vi "Get Access Token.vi"(8 "Error In (No Error)":errorcluster) -> (1 "token response (JSON)":string, 2 "access token":string caption="<JSON>Item")   [LabVIEW 2019, in "Useful OAuth VIs.lvlib"]
uses:
  Useful OAuth VIs.lvlib
  e7adaa82-728e-4af2-911a-35986e5cd437.vi
  2f0a06cf-a99b-4825-b433-179a9c98a469.vi
  <vilib>/JDP Science/JSONtext/Find Item.vi
  <vilib>/JDP Science/JSONtext/String Subset.vi
  globals.vi
  <vilib>/httpClient/POSTBuffer.vi
  <vilib>/JDP Science/JSONtext/Parsing/Parse Full Path or Item Name.vi
  <vilib>/JDP Science/JSONtext/Next JSON Value.vi
  <vilib>/JDP Science/JSONtext/support/Error Cluster From Code.vi
  <vilib>/JDP Science/JSONtext/Offset/Find Item Locations by Path.vi
  <vilib>/JDP Science/JSONtext/JSON text to Variant.vi
  <vilib>/JDP Science/JSONtext/LVClass Serializer/JSONtext LVClass Serializer.lvclass
  <vilib>/httpClient/LabVIEWHTTPClient.lvlib
  <vilib>/wsapi/NI_WebServices.lvlib
panel:
  out "error out":errorcluster
  in  "Redirect URI":string="http://localhost:8001/OAuth/Redirect"
  in  "Client Secret":string="Tx~D4BO32ip_x~_salD8.nHFyC7XIXCKuI"
  in  "Scopes (separated by single space)":string="offline_access Notes.ReadWrite"
  in  "Client ID":string="6224e1bc-8db0-4ef6-9504-7e49f93fdd78"
  in  "Tenant Type":string="organizations"
  out "Request body":string
  out "Request URI":string
  out "headers":string
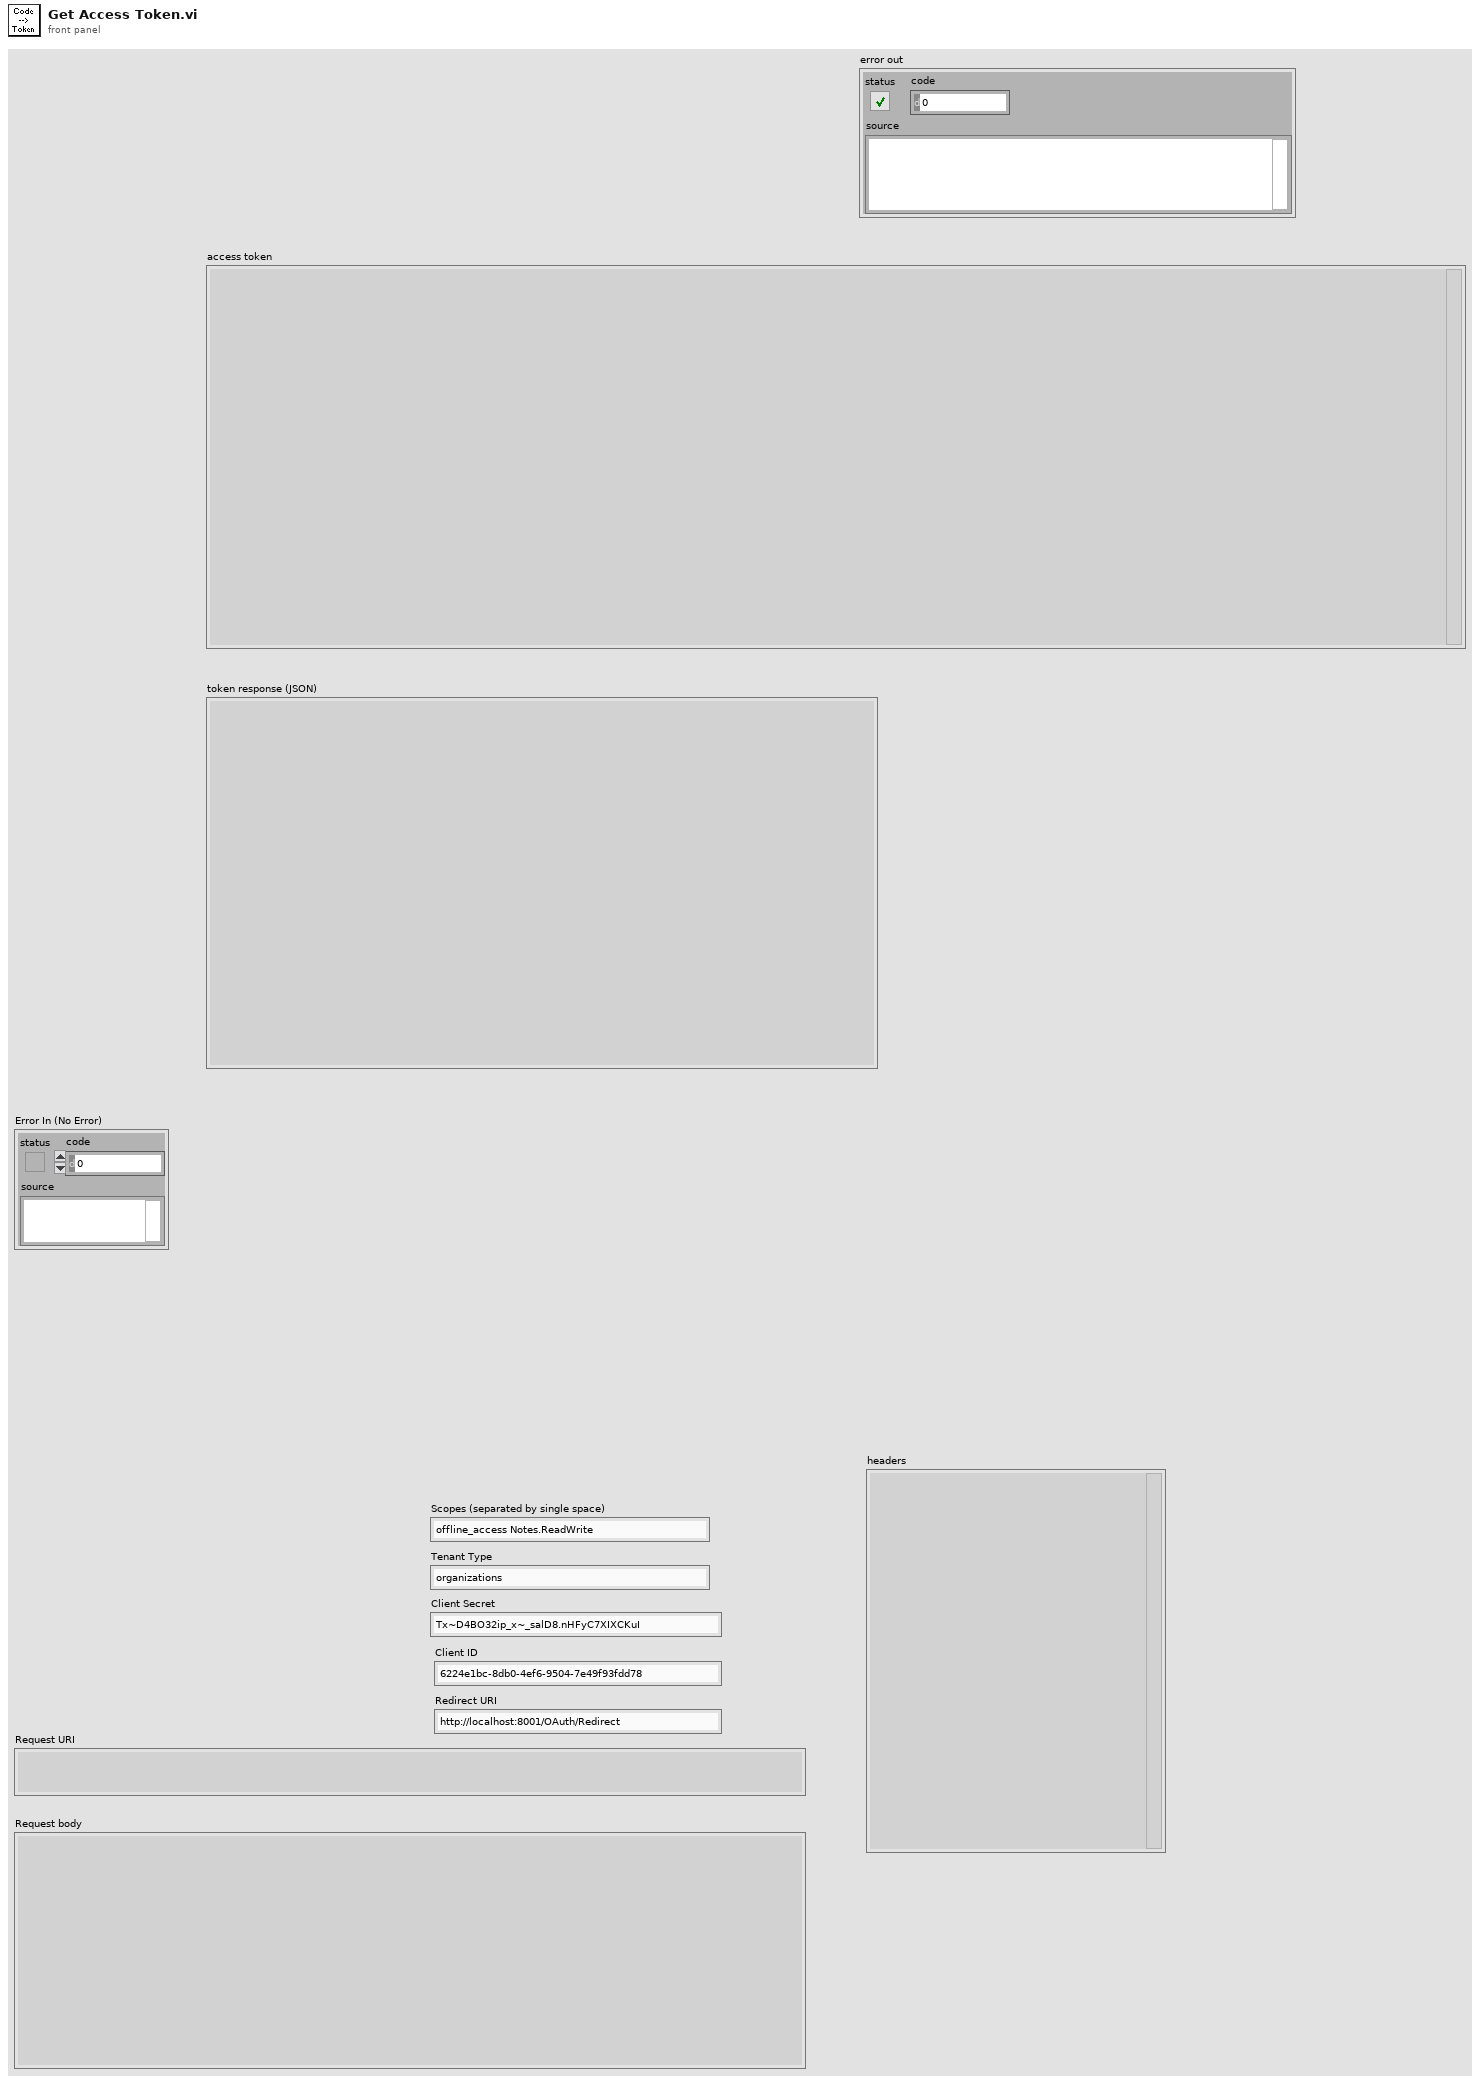
[diagram p1: front panel]
types:
  T1 = typedef "LabVIEWHTTPClient.lvlib/ClientHandle.ctl" = refnum<k1>
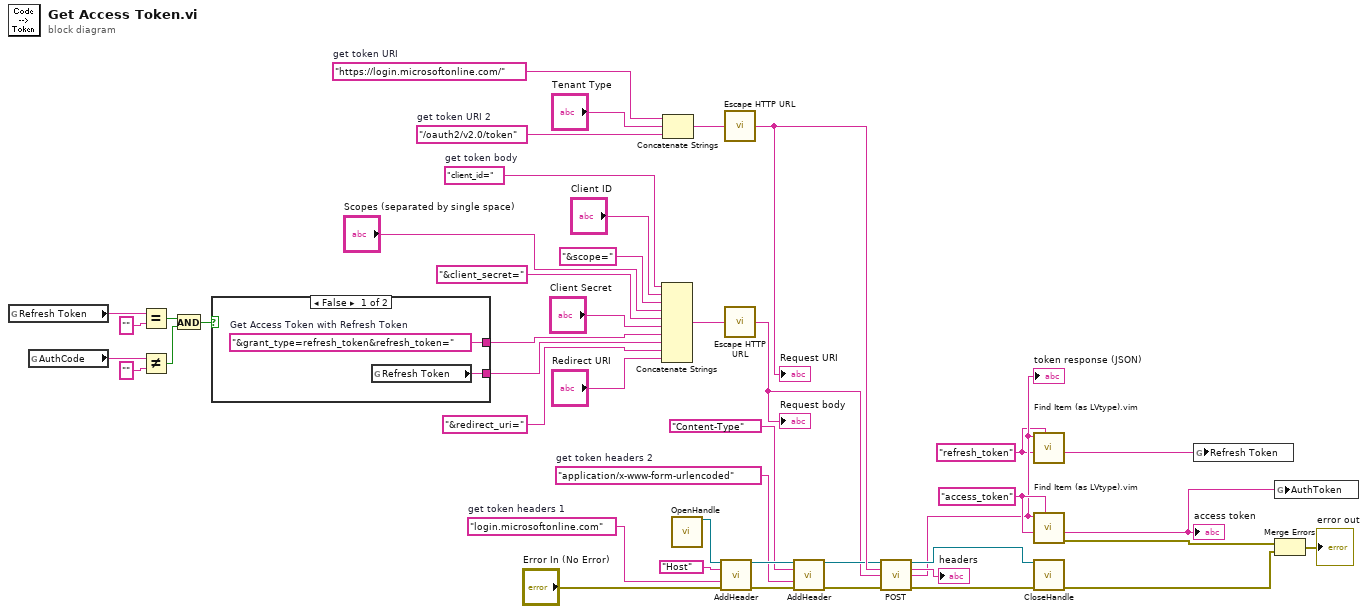
[diagram p0: block diagram]
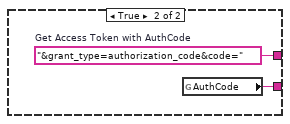
[diagram p2: hidden frame]
diagram:
  w9 = "refresh_token" ("$Path or Item Name")
  w30 = "access_token" ("key")
  w34 = "application/x-www-form-urlencoded"  # get token headers 2
  w36 = "login.microsoftonline.com"  # get token headers 1
  w43 = "/oauth2/v2.0/token"  # get token URI 2
  w41 = "https://login.microsoftonline.com/"  # get token URI
  w32 = "client_id="  # get token body
  n1 = global read "globals.vi" "Refresh Token"() -> (w4:string)
  n2 = global read "globals.vi" "AuthCode"() -> (w7:string)
  n3 = Equal?(x=w4, y="") -> (x = y?=w1:bool)
  n4 = Not Equal?(x=w7, y="") -> (x != y?=w3:bool)
  n5 = And(x=w1, y=w3) -> (x .and. y?=w5:bool)
  n6 = case shown="False" w5 {
    tunnel: [w47 w49] -> w28
    tunnel: [w46 w48] -> w12
    frame False {
      w47 = "&grant_type=refresh_token&refresh_token="  # Get Access Token with Refresh Token
      n7 = global read "globals.vi" "Refresh Token"() -> (w46:string)
    }
    frame True {
      w49 = "&grant_type=authorization_code&code="  # Get Access Token with AuthCode
      n8 = global read "globals.vi" "AuthCode"() -> (w48:string)
    }
  }
  n9 = Concatenate Strings(w32, "Client ID", "&scope=" ("string"), "Scopes (separated by single space)", "&client_secret=" ("string"), "Client Secret", w28, w12, "&redirect_uri=" ("string"), "Redirect URI") -> (w27:string)
  n10 = Concatenate Strings(w41, "Tenant Type", w43) -> (w42:string)
  n11 = call <vilib>:"OpenHandle.vi"() -> ("client handle out"=w21:T1)  [unwired: 14 in, 1 out]
  n12 = call <vilib>:"AddHeader.vi"("client handle"=w21, "header"="Host", "value"=w36, "error in (no error)"="Error In (No Error)") -> ("client handle out"=w45:T1, "error out"=w44:errorcluster)  [unwired: 10 in]
  n13 = call <vilib>:"Escape HTTP URL.vi"("unescaped string in"=w42) -> ("escaped string out"=w40:string)
  "Request URI" <- w40
  n14 = call <vilib>:"Escape HTTP URL.vi"("unescaped string in"=w27) -> ("escaped string out"=w26:string)
  "Request body" <- w26
  n15 = call <vilib>:"AddHeader.vi"("client handle"=w45, "header"="Content-Type", "value"=w34, "error in (no error)"=w44) -> ("client handle out"=w33:T1, "error out"=w38:errorcluster)  [unwired: 10 in]
  n16 = call-poly <vilib>:"POST.vi"("client handle"=w33, "url"=w40, "buffer"=w26, "error in (no error)"=w38) -> ("client handle out"=w20:T1, "headers"=→"headers":string, "body"=w10:string, "error out"=w18:errorcluster)  [unwired: 8 in]
  "token response (JSON)" <- w10
  n17 = call "Find Item (as LVtype).vim"("$Path or Item Name"=w9, "Data Type and Default Value"=w9, "JSON"=w10) -> ("Data"=w8:string)  [unwired: 5 in, 3 out]
  n18 = call "Find Item (as LVtype).vim"("$Path or Item Name"=w30, "Data Type and Default Value"=w30, "JSON"=w10) -> ("error out"=w29:errorcluster, "Data"=w11:string)  [unwired: 5 in, 2 out]
  "access token" <- w11
  n19 = call <vilib>:"CloseHandle.vi"("client handle"=w20, "error in (no error)"=w18) -> ("error out"=w19:errorcluster)  [unwired: 13 in]
  n20 = global write "globals.vi" "Refresh Token"(w8) -> ()
  n21 = global write "globals.vi" "AuthToken"(w11) -> ()
  n22 = Merge Errors(w29, w19) -> (→"error out":errorcluster)
